vi "Get Metadata.vi"(7 "error in":errorcluster, 9 "measurement control path":path, 10 "measurement plugin service in":refnum<class "Measurement Plugin Service.lvclass">) -> (0 "error out":errorcluster, 2 "metadata value":T2(array[cluster]), 3 "measurement plugin service out":refnum<class "Measurement Plugin Service.lvclass">)   [LabVIEW 2020, in "MeasurementLink Measurement Server.lvlib"]
uses:
  MeasurementLink Measurement Server.lvlib
  TypeDefs/Parameter_AnnotationsEntry.ctl
  Measurement Plugin Service/Measurement Plugin Service.lvclass
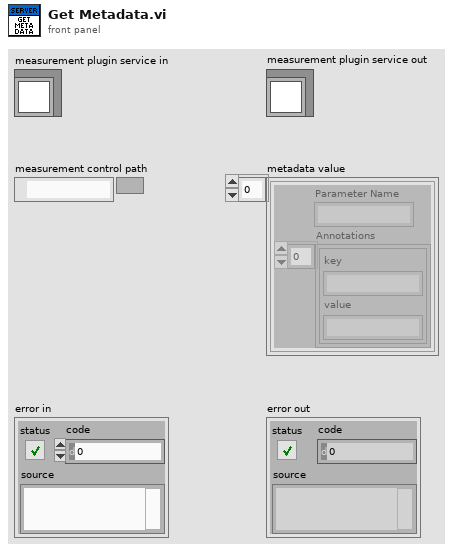
[diagram p1: front panel]
types:
  T1 = typedef "MeasurementLink Measurement Server.lvlib/Parameter_AnnotationsEntry.ctl" = cluster{"key":string, "value":string}
  T2 = cluster{"Parameter Name":string, "Annotations":T1[]}[]
  T3 = typedef "MeasurementLink Measurement Server.lvlib/Parameter Type Specialization.ctl" = cluster{"Parameter Name":string, "Type Specialization":T4, "Annotations":cluster{"Key":T5, "Value":string}[]}
  T4 = typedef "MeasurementLink Measurement Server.lvlib/Type Specialization.ctl" = enum16{"none", "pin", "path", "enum"}
  T5 = typedef "MeasurementLink Measurement Server.lvlib/Type Specialization Key.ctl" = enum16{"none", "pin.instrument_type", "enum.values"}
  T6 = cluster{"Parameter Name":string, "Annotations":T1[]}
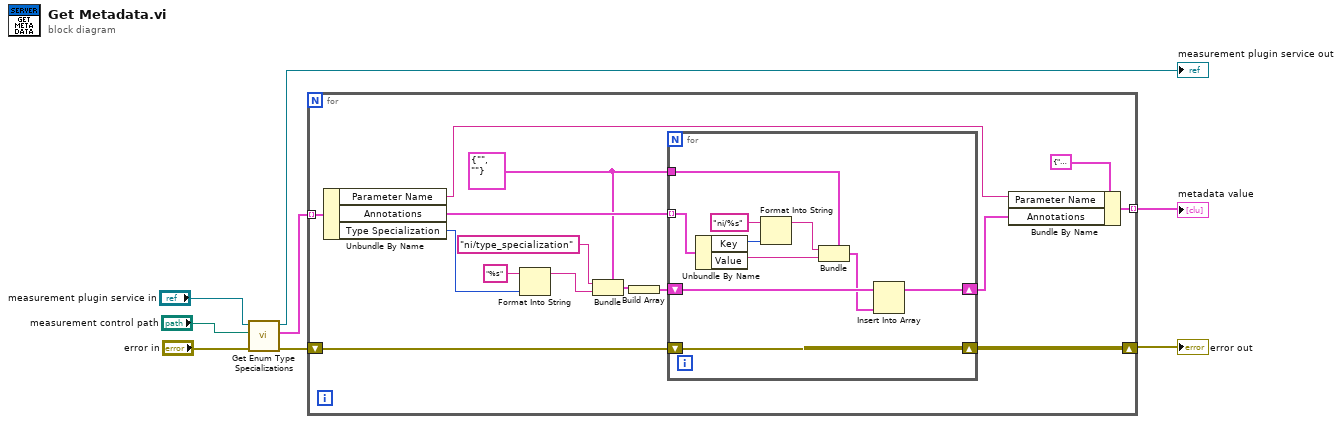
[diagram p0: block diagram]
diagram:
  n1 = call "Get Enum Type Specializations.vi"("error in"="error in", "measurement control path"="measurement control path", "measurement plugin service in"="measurement plugin service in") -> ("error out"=w5:errorcluster, "type specializations"=w6:T3[], "measurement plugin service out"=→"measurement plugin service out":refnum<class "Measurement Plugin Service.lvclass">)  [unwired: 6 in]
  n2 = for {
    tunnel: w6 -> [w23] mode=indexing
    shift-right: [w19] -> w7
    shift-left: w5 -> [w20]
    tunnel: [w21] -> w8 mode=indexing
    w9 = T1 {"key"="", "value"=""} ("Parameter_AnnotationsEntry")
    n3 = Unbundle By Name(w23) -> ("Parameter Name"=w10:string, "Annotations"=w14:cluster{"Key":T5, "Value":string}[], "Type Specialization"=w18:T4)
    n4 = Format Into String(format string="%s", w18) -> (resulting string=w16:string)  [unwired: 2 in, 1 out]
    n5 = Bundle(cluster=w9, "key"="ni/type_specialization" ("Value"), "value"=w16) -> (w11:T1)
    n6 = Build Array(w11) -> (w12:T1[])
    n7 = for {
      shift-right: [w33] -> w19
      shift-left: w20 -> [w33]
      tunnel: w14 -> [w32] mode=indexing
      shift-right: [w25] -> w13
      shift-left: w12 -> [w27]
      tunnel: w9 -> [w24]
      n8 = Unbundle By Name(w32) -> ("Key"=w30:T5, "Value"=w28:string)
      n9 = Format Into String(format string="ni/%s", w30) -> (resulting string=w29:string)  [unwired: 2 in, 1 out]
      n10 = Bundle(cluster=w24, "key"=w29, "value"=w28) -> (w26:T1)
      n11 = Insert Into Array(array=w27, new element=w26) -> (w25:T1[])  [unwired: 1 in]
    }
    n12 = Bundle By Name(cluster=T6 {"Parameter Name"="", "Annotations"=[{"key"="", "value"=""}]} ("Cluster"), "Parameter Name"=w10, "Annotations"=w13) -> (w21:T6)
  }
  "error out" <- w7
  "metadata value" <- w8
